vi "Pre Launch Init.vi"(11 "Cli in":refnum<class "Cli.lvclass">) -> (0 "error out":errorcluster, 3 "Cli out":refnum<class "Cli.lvclass">)   [LabVIEW 2022 SP3, in "Cli.lvlib" / "Cli.lvclass"]
doc: "(<B>Filename</B>: Actor Framework.lvlib:Actor.lvclass:Pre Launch Init.vi)\n\nDefines behavior that occurs after the Launch Actor method is invoked but before the actor's Actor Core method begins running.\n\nThe Pre Launch Init method is guaranteed to finish before the Launch Actor method returns to its caller and before the actor itself receives any messages. Any references that the Pre Launch Init method obtains are guaranteed to have the same lifetime as the actor itself. Any errors that the Pre Launch Init method returns will abort the launch.\n\nBy default, this method does nothing. A descendant class may override it to define behavior."
uses:
  Cli.lvclass
  Cli.lvclass/Cli.ctl
  LoggingActor/Source/LoggingActor/LoggingActor/LoggingActor.lvclass
  ArgumentParser/Source/ArgumentParser/ArgumentParser.lvclass
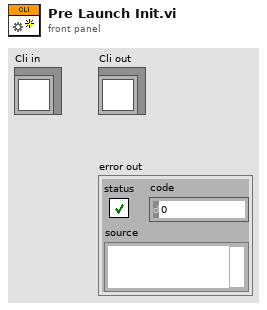
[diagram p1: front panel]
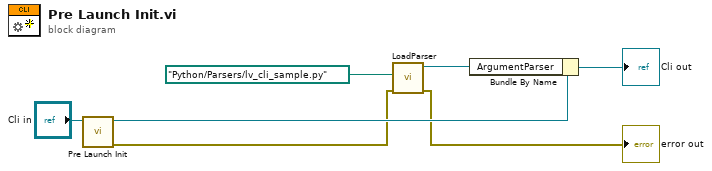
[diagram p0: block diagram]
diagram:
  n1 = call-parent "Pre Launch Init.vi"("LoggingActor in"="Cli in") -> ("error out"=w2:errorcluster, "LoggingActor out"=w6:refnum<class "Cli.lvclass">)  [unwired: 9 in]
  n2 = call "LoadParser.vi"("error in (no error)"=w2, "ParserPath"=path "Python/Parsers/lv_cli_sample.py") -> ("error out"=→"error out":errorcluster, "ArgumentParser"=w3:refnum<class "ArgumentParser.lvclass">)  [unwired: 8 in]
  n3 = Bundle By Name(cluster=w6, "ArgumentParser"=w3) -> (→"Cli out":refnum<class "Cli.lvclass">)
